vi "Charger_Wake-Up IPG.vi"(6 "error in":errorcluster, 7 "Pulse Duration (3 s)":dbl[unit]=3.0, 9 "Charger":T1={"address"="COM17", "position"=2, "setpoint"=7500.0} {"setpoint" min=0.0 max=20000.0 step=100.0; "position" min=0 max=5 step=1}) -> (0 "error out":errorcluster)   [LabVIEW 2010]
doc: "This function wakes-up a single IPG with a 3-second charge pulse."
uses:
  Charger_Input Control.ctl
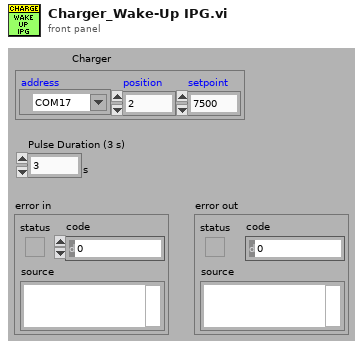
[diagram p1: front panel]
types:
  T1 = typedef "Charger_Input Control.ctl" = cluster{"address":refnum<visa-resource-name>, "position":i32, "setpoint":dbl}
  T2 = enum16{"Disable", "Enable", "Update", "Get Info"}
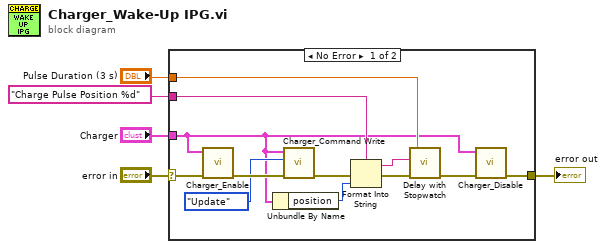
[diagram p0: block diagram]
diagram:
  n1 = case shown="No Error" "error in" {
    selector: "error in" -> [w16 w18]
    tunnel: [w6 w18] -> w5
    tunnel: "Charge Pulse Position %d" ("window title") -> [w10 _]
    tunnel: "Pulse Duration (3 s)" -> [w9 _]
    tunnel: "Charger" -> [w8 _]
    frame No Error {
      n2 = call "Charger_Enable.vi"("error in"=w16, "Charger"=w8) -> ("error out"=w15:errorcluster)  [unwired: 7 in]
      n3 = Unbundle By Name(w8) -> ("position"=w7:i32)
      n4 = call "Charger_Command Write.vi"("error in"=w15, "Command"=T2."Update", "Charger"=w8) -> ("error out"=w13:errorcluster)  [unwired: 5 in, 1 out]
      n5 = Format Into String(format string=w10, error in=w13, w7) -> (resulting string=w11:string, error out=w12:errorcluster)  [unwired: 1 in]
      n6 = call "Delay with Stopwatch.vi"("error in"=w12, "window title"=w11, "delay"=w9) -> ("error out"=w17:errorcluster)  [unwired: 4 in]
      n7 = call "Charger_Disable.vi"("error in"=w17, "Charger"=w8) -> ("error out"=w6:errorcluster)  [unwired: 7 in]
    }
    frame Error {
    }
  }
  "error out" <- w5
